vi "定时启动 (子VI).vi"   [LabVIEW 2016, in "斯坦道CODMn.lvlib"]
types:
  T1 = cluster{"测量模式":enum16{"水样测量", "标样核查", "零点核查", "跨度核查", "空白测试", "加标回收", "平行样", "校零", "校标"}}
  T2 = cluster{"仪器测试类型":enum16{"水样测试", "零点核查", "标样核查", "空白测试", "跨度核查", "加标回收", "平行样", "校零", "校标"}, "周期设置类型":enum16{"定点启动", "间隔启动"}, "定时功能启用":bool, "定时间隔":dbl, "24H周期设置":bool[]}
  T3 = typedef "LVDateTimeRec.ctl" = cluster{"秒数的小数部分":dbl, "秒":i32, "分":i32, "时":i32, "日":i32, "月":i32, "年":i32, "天数（周）":i32, "天数（年）":i32, "DST":i32}
  T4 = enum16{"水样测试", "零点核查", "标样核查", "空白测试", "跨度核查", "加标回收", "平行样", "校零", "校标"}
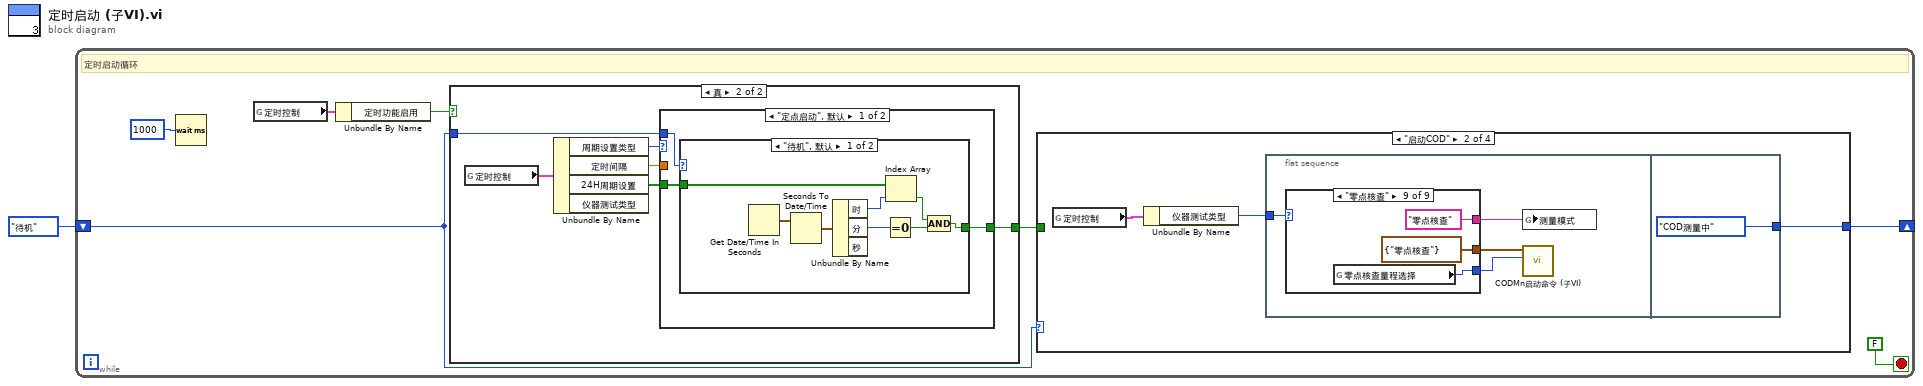
[diagram p0: block diagram]
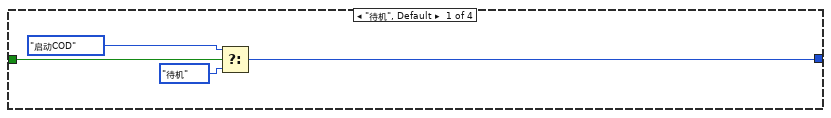
[diagram p2: hidden frame]
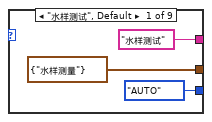
[diagram p3: hidden frame]
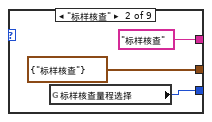
[diagram p4: hidden frame]
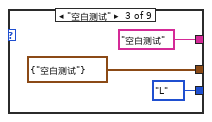
[diagram p5: hidden frame]
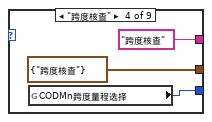
[diagram p6: hidden frame]
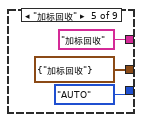
[diagram p7: hidden frame]
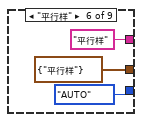
[diagram p8: hidden frame]
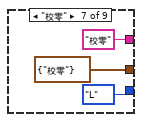
[diagram p9: hidden frame]
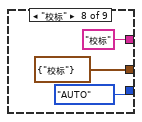
[diagram p10: hidden frame]
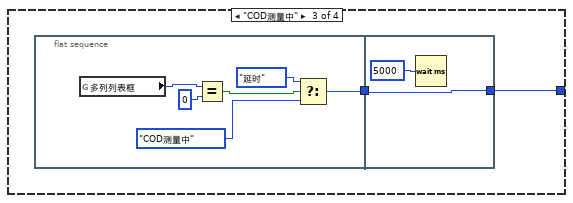
[diagram p11: hidden frame]
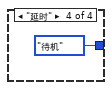
[diagram p12: hidden frame]
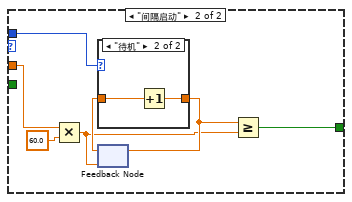
[diagram p15: hidden frame]
diagram:
  n1 = while {
    shift-right: [w6] -> _
    shift-left: enum16{"待机", "启动COD", "COD测量中", "延时"}."待机" -> [w5]
    stop <- FALSE stop-if-true
    # "定时启动循环"
    n2 = Wait (ms)(milliseconds to wait=u32 1000 ("等待时间（毫秒）")) -> ()  [unwired: 1 out]
    n3 = global read "CODMn断电保存全局变量.vi" "定时控制"() -> (w3:T2)
    n4 = Unbundle By Name(w3) -> ("定时功能启用"=w2:bool)
    n5 = case shown="真" w2 {
      tunnel: w5 -> [_ w61]
      tunnel: [_ w60] -> w4
      frame False {
      }
      frame True {
        n6 = global read "CODMn断电保存全局变量.vi" "定时控制"() -> (w59:T2)
        n7 = Unbundle By Name(w59) -> ("周期设置类型"=w62:enum16{"定点启动", "间隔启动"}, "定时间隔"=w63:dbl, "24H周期设置"=w64:bool[])  [unwired: 1 out]
        n8 = case shown="\"定点启动\", 默认" w62 {
          tunnel: w63 -> [_ w79]
          tunnel: w64 -> [w67 _]
          tunnel: w61 -> [w65 w82]
          tunnel: [w66 w77] -> w60
          frame "定点启动", Default {
            n9 = case shown="\"待机\", 默认" w65 {
              tunnel: w67 -> [w73 _]
              tunnel: [w68 _] -> w66
              frame "待机", Default {
                n10 = Get Date/Time In Seconds() -> (seconds since 1Jan1904=w75:timestamp)
                n11 = Seconds To Date/Time(time stamp (now)=w75) -> (date time rec=w74:T3)  [unwired: 1 in]
                n12 = Unbundle By Name(w74) -> ("时"=w72:i32, "分"=w71:i32)  [unwired: 1 out]
                n13 = Equal To 0?(x=w71) -> (x = 0?=w69:bool)
                n14 = Index Array(array=w73, index=w72) -> (element=w70:bool)
                n15 = Compound Arithmetic op=AND ("复合运算")(w70, w69) -> (w68:bool)
              }
              frame "启动COD" {
              }
            }
          }
          frame "间隔启动" {
            n16 = Multiply(x=w79, y=60.0) -> (x*y=w76:dbl)
            n17 = feedback #1(w76) -> (w81:dbl)
            n18 = case shown="\"待机\"" w82 {
              tunnel: w81 -> [_ w84]
              tunnel: [_ w83] -> w80
              frame Default {
              }
              frame "待机" {
                n19 = Increment(x=w84) -> (x+1=w83:dbl)
              }
            }
            n20 = feedback-in #1(w80) -> ()
            n21 = Greater Or Equal?(x=w80, y=w76) -> (x >= y?=w77:bool)
          }
        }
      }
    }
    n22 = case shown="\"启动COD\"" w5 {
      tunnel: [w9 w15 w49 enum16{"待机", "启动COD", "COD测量中", "延时"}."待机"] -> w6
      tunnel: w4 -> [w12 _ _ _]
      frame "待机", Default {
        n23 = Select(t=enum16{"待机", "启动COD", "COD测量中", "延时"}."启动COD", s=w12, f=enum16{"待机", "启动COD", "COD测量中", "延时"}."待机") -> (s? t:f=w9:enum16{"待机", "启动COD", "COD测量中", "延时"})
      }
      frame "启动COD" {
        n24 = global read "CODMn断电保存全局变量.vi" "定时控制"() -> (w13:T2)
        n25 = Unbundle By Name(w13) -> ("仪器测试类型"=w14:T4)
        n26 = flat-sequence {
          tunnel: w14 -> [w19]
          tunnel: [enum16{"待机", "启动COD", "COD测量中", "延时"}."COD测量中"] -> w15
          frame #0 {
            n27 = case shown="\"零点核查\"" w19 {
              tunnel: [T1 {"测量模式"=enum."水样测量"} ("启动测量模式") T1 {"测量模式"=enum."标样核查"} ("启动测量模式") T1 {"测量模式"=enum."空白测试"} ("启动测量模式") T1 {"测量模式"=enum."跨度核查"} ("启动测量模式") T1 {"测量模式"=enum."加标回收"} ("启动测量模式") T1 {"测量模式"=enum."平行样"} ("启动测量模式") T1 {"测量模式"=enum."校零"} ("启动测量模式") T1 {"测量模式"=enum."校标"} ("启动测量模式") T1 {"测量模式"=enum."零点核查"} ("启动测量模式")] -> w18
              tunnel: ["水样测试" ("测量模式") "标样核查" ("测量模式") "空白测试" ("测量模式") "跨度核查" ("测量模式") "加标回收" ("测量模式") "平行样" ("测量模式") "校零" ("测量模式") "校标" ("测量模式") "零点核查" ("测量模式")] -> w17
              tunnel: [enum32{"H", "L", "AUTO"}."AUTO" ("CODMn跨度量程选择") w23 enum32{"H", "L", "AUTO"}."L" ("CODMn跨度量程选择") w29 enum32{"H", "L", "AUTO"}."AUTO" ("CODMn跨度量程选择") enum32{"H", "L", "AUTO"}."AUTO" ("CODMn跨度量程选择") enum32{"H", "L", "AUTO"}."L" ("CODMn跨度量程选择") enum32{"H", "L", "AUTO"}."AUTO" ("CODMn跨度量程选择") w44] -> w16
              frame "水样测试", Default {
              }
              frame "标样核查" {
                n28 = global read "CODMn断电保存全局变量.vi" "标样核查量程选择"() -> (w23:enum32{"H", "L", "AUTO"})
              }
              frame "空白测试" {
              }
              frame "跨度核查" {
                n29 = global read "CODMn断电保存全局变量.vi" "CODMn跨度量程选择"() -> (w29:enum32{"H", "L", "AUTO"})
              }
              frame "加标回收" {
              }
              frame "平行样" {
              }
              frame "校零" {
              }
              frame "校标" {
              }
              frame "零点核查" {
                n30 = global read "CODMn断电保存全局变量.vi" "零点核查量程选择"() -> (w44:enum32{"H", "L", "AUTO"})
              }
            }
            n31 = global write "COD测量模式全局.vi" "测量模式"(w17) -> ()
            n32 = call "CODMn启动命令 (子VI).vi"("CODMn量程切换"=w16, "启动测量模式"=w18) -> ()  [unwired: 10 in]
          }
          frame #1 {
          }
        }
      }
      frame "COD测量中" {
        n33 = flat-sequence {
          tunnel: [w50] -> w48
          tunnel: [w57] -> w49
          tunnel: w48 -> [w57]
          frame #0 {
            n34 = global read "运行时序全局变量.vi" "多列列表框"() -> (w55:i32)
            n35 = Equal?(x=w55, y=0) -> (x = y?=w53:bool)
            n36 = Select(t=enum16{"待机", "启动COD", "COD测量中", "延时"}."延时", s=w53, f=enum16{"待机", "启动COD", "COD测量中", "延时"}."COD测量中") -> (s? t:f=w50:enum16{"待机", "启动COD", "COD测量中", "延时"})
          }
          frame #1 {
            n37 = Wait (ms)(milliseconds to wait=u32 5000 ("等待时间（毫秒）")) -> ()  [unwired: 1 out]
          }
        }
      }
      frame "延时" {
      }
    }
  }
